vi "sandbox.vi"() -> ()   [LabVIEW 2019, in "Instrument UI.Lockin.lvclass"]
uses:
  Instrument UI.Lockin.lvclass
  Instrument.DAQ/Typedefs/Set State-enum.ctl
  Instrument.DAQ/Instrument.DAQ.lvclass
panel:
  out "delimited string":string
  out "output 1":T1
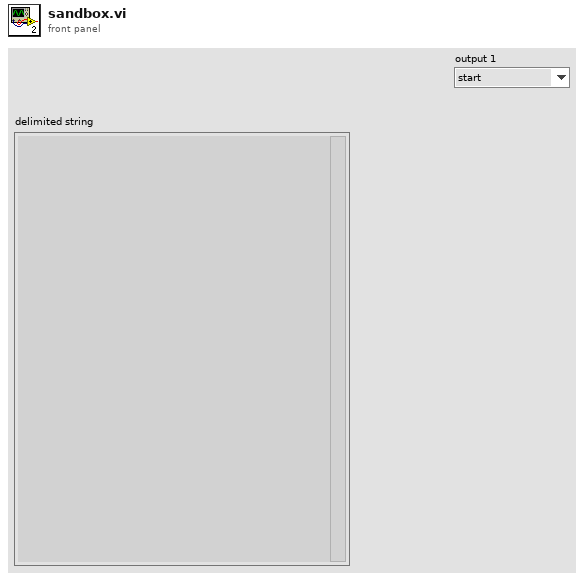
[diagram p1: front panel]
types:
  T1 = typedef "Instrument.DAQ.lvclass/Set State-enum.ctl" = enum16{"start", "stop", "reset", "start sweep", "stop sweep"}
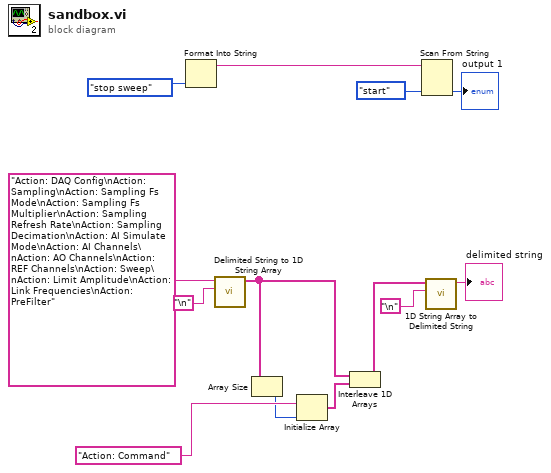
[diagram p0: block diagram]
diagram:
  n1 = Format Into String(Set_State-enum."stop sweep" ("State")) -> (resulting string=w11:string)  [unwired: 3 in, 1 out]
  n2 = call <vilib>:"Delimited String to 1D String Array.vi"("delimiter"="\n", "delimited string"="Action: DAQ Config\nAction: Sampling\nAction: Sampling Fs Mode\nAction: Sampling Fs Multiplier\nAction: Sampling Refresh Rate\nAction: Sampling Decimation\nAction: AI Simulate Mode\nAction: AI Channels\nAction: AO Channels\nAction: REF Channels\nAction: Sweep\nAction: Limit Amplitude\nAction: Link Frequencies\nAction: PreFilter" ("State(s) in Front (\"\")")) -> ("string array"=w3:string[])  [unwired: 9 in]
  n3 = Array Size(array=w3) -> (size(s)=w6:i32)
  n4 = Initialize Array("Action: Command", w6) -> (w5:string[])
  n5 = Interleave 1D Arrays(w3, w5) -> (w4:string[])
  n6 = Scan From String(input string=w11, default 1=Set_State-enum."start" ("State")) -> (output 1=→"output 1":T1)  [unwired: 3 in, 3 out]
  n7 = call <vilib>:"1D String Array to Delimited String.vi"("delimiter"="\n", "string array"=w4) -> ("delimited string"=→"delimited string":string)  [unwired: 9 in]
